vi "CRYTrigger advanced.vi"(0 "N sample":i32, 1 "N points":i32, 5 "Slope":u32(slide), 7 "Signal":dbl[](array[numeric]), 9 "Pretrigger ms":dbl format="%.6f", 11 "Trigger level (counts)":i32 format="%.3f", 12 "dt":dbl format="%.6f", 13 "Free run":bool, 15 "Reset buffer":bool) -> (4 "Triggered signal":dbl[](array[numeric]), 6 "Triggered":bool)   [LabVIEW 2013]
panel:
  out "x+y 2":i32
  out "x+y":i32
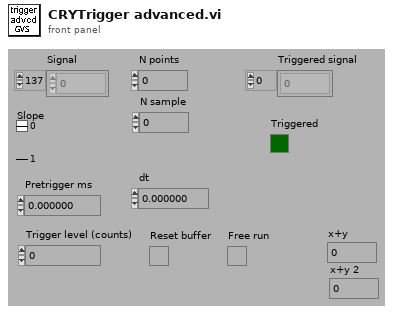
[diagram p1: front panel]
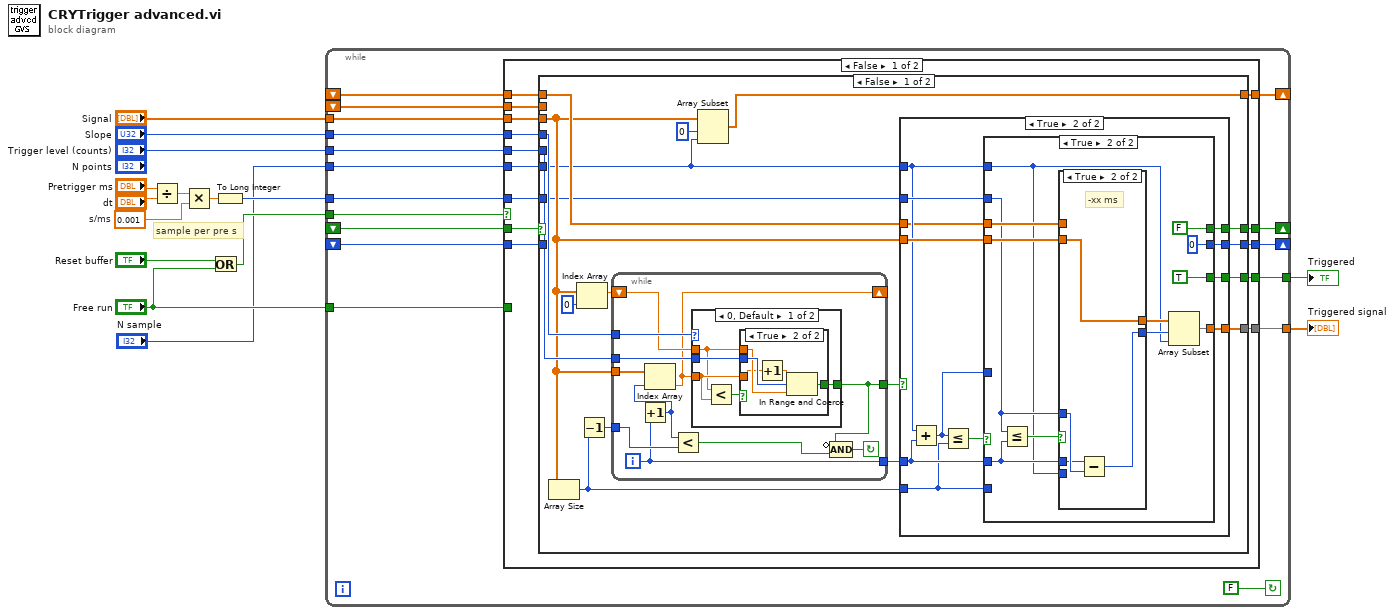
[diagram p0: block diagram]
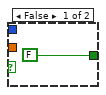
[diagram p2: hidden frame]
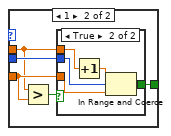
[diagram p3: hidden frame]
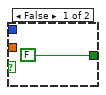
[diagram p4: hidden frame]
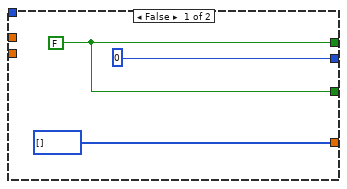
[diagram p5: hidden frame]
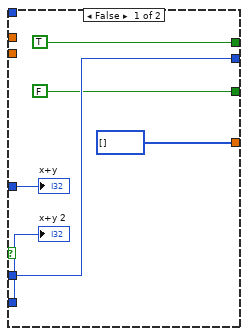
[diagram p6: hidden frame]
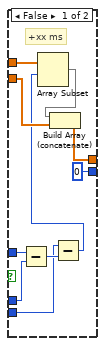
[diagram p7: hidden frame]
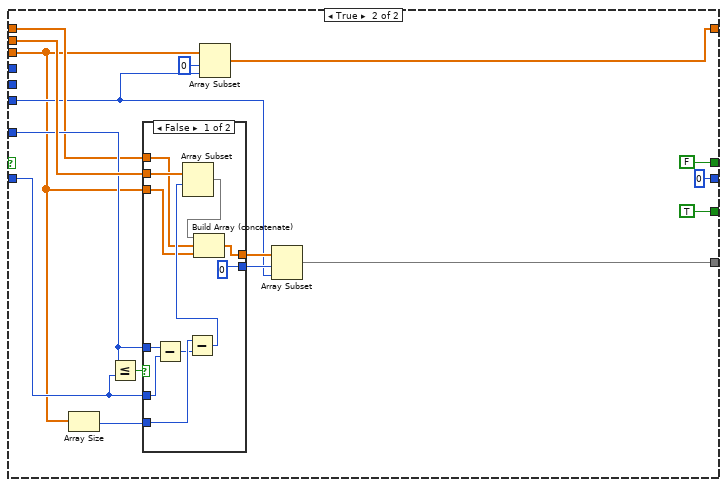
[diagram p8: hidden frame]
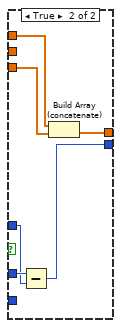
[diagram p9: hidden frame]
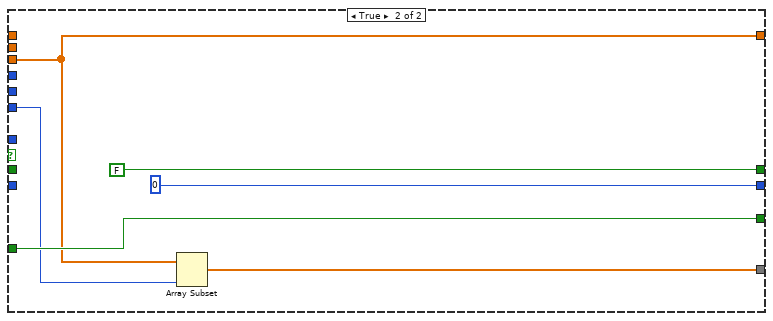
[diagram p10: hidden frame]
diagram:
  w10 = 0.001  # s/ms
  # "sample per pre s"
  n1 = Divide(x="Pretrigger ms", y="dt") -> (x/y=w9:dbl)
  n2 = Multiply(x=w9, y=w10) -> (x*y=w8:dbl)
  n3 = Or(x="Reset buffer", y="Free run") -> (x .or. y?=w4:bool)
  n4 = To Long Integer(number=w8) -> (32bit integer=w7:i32)
  n5 = while {
    tunnel: "Free run" -> [w19]
    shift-left: _ -> [w20]
    tunnel: w7 -> [w21]
    tunnel: "N sample" -> [w22]
    tunnel: "Trigger level (counts)" -> [w23]
    tunnel: "Slope" -> [w24]
    shift-left: _ -> [w25]
    shift-right: [w26] -> _
    tunnel: [w27] -> w2
    tunnel: [w28] -> w15
    tunnel: "Signal" -> [w16]
    tunnel: w4 -> [w32]
    shift-left: _ -> [w29]
    shift-right: [w30] -> _
    shift-left: _ -> [w17]
    shift-right: [w31] -> _
    stop <- FALSE continue-if-true
    n6 = case shown="False" w32 {
      tunnel: [w37 w180] -> w31
      tunnel: w16 -> [w44 w180]
      tunnel: [w40 FALSE] -> w30
      tunnel: w29 -> [w46 _]
      tunnel: w17 -> [w45 _]
      tunnel: [w39 w181] -> w28
      tunnel: [w41 w179] -> w27
      tunnel: [w38 0] -> w26
      tunnel: w25 -> [w33 _]
      tunnel: w24 -> [w43 _]
      tunnel: w23 -> [w42 _]
      tunnel: w22 -> [w36 w178]
      tunnel: w21 -> [w35 _]
      tunnel: w20 -> [w34 _]
      tunnel: w19 -> [_ w181]
      frame False {
        n7 = case shown="False" w46 {
          tunnel: w45 -> [w53 w149]
          tunnel: w44 -> [w52 w145]
          tunnel: w43 -> [w62 _]
          tunnel: w42 -> [w61 _]
          tunnel: [w59 w150] -> w41
          tunnel: [w58 FALSE] -> w40
          tunnel: [w57 TRUE] -> w39
          tunnel: [w56 0] -> w38
          tunnel: [w51 w146] -> w37
          tunnel: w36 -> [w50 w148]
          tunnel: w35 -> [w48 w151]
          tunnel: w34 -> [_ w153]
          tunnel: w33 -> [_ w154]
          frame False {
            n8 = Array Size(array=w52) -> (size(s)=w54:i32)
            n9 = Index Array(array=w52, index=0) -> (element=w63:dbl)
            n10 = Decrement(x=w54) -> (x-1=w64:i32)
            n11 = while {
              tunnel: [w65] -> w55
              tunnel: [w66] -> w60
              tunnel: w61 -> [w72]
              tunnel: w62 -> [w74]
              shift-left: w63 -> [w73]
              shift-right: [w71] -> _
              tunnel: w64 -> [w69]
              tunnel: w52 -> [w75]
              i -> [w65]
              stop <- w67 continue-if-true
              n12 = Increment(x=w65) -> (x+1=w70:i32)
              n13 = Index Array(array=w75, index=w70) -> (element=w71:dbl)
              n14 = Less?(x=w70, y=w69) -> (x < y?=w68:bool)
              n15 = case shown="0, Default" w74 {
                tunnel: w73 -> [w77 w88]
                tunnel: w72 -> [w79 w90]
                tunnel: w71 -> [w78 w89]
                tunnel: [w76 w87] -> w66
                frame 0, Default {
                  n16 = Less?(x=w77, y=w78) -> (x < y?=w80:bool)
                  n17 = case shown="True" w80 {
                    tunnel: w79 -> [_ w86]
                    tunnel: w78 -> [_ w83]
                    tunnel: w77 -> [_ w85]
                    tunnel: [FALSE w84] -> w76
                    frame False {
                    }
                    frame True {
                      n18 = Increment(x=w83) -> (x+1=w82:dbl)
                      n19 = In Range and Coerce(upper limit=w82, x=w86, lower limit=w85) -> (In Range?=w84:bool)  [unwired: 1 out]
                    }
                  }
                }
                frame 1 {
                  n20 = Greater?(x=w88, y=w89) -> (0:w91:bool)
                  n21 = case shown="True" w91 {
                    tunnel: w90 -> [_ w97]
                    tunnel: w89 -> [_ w95]
                    tunnel: w88 -> [_ w94]
                    tunnel: [FALSE w96] -> w87
                    frame False {
                    }
                    frame True {
                      n22 = Increment(x=w94) -> (x+1=w93:dbl)
                      n23 = In Range and Coerce(upper limit=w93, x=w97, lower limit=w95) -> (In Range?=w96:bool)  [unwired: 1 out]
                    }
                  }
                }
              }
              n24 = Compound Arithmetic op=AND(invert w66, w68) -> (w67:bool)
            }
            n25 = Array Subset(array=w52, index=0, length=w50) -> (w51:dbl[])
            n26 = case shown="True" w60 {
              tunnel: [i32[] [] ("Triggered signal") w107] -> w59
              tunnel: [w99 w111] -> w58
              tunnel: [w99 w108] -> w57
              tunnel: [0 w110] -> w56
              tunnel: w50 -> [_ w104]
              tunnel: w55 -> [_ w109]
              tunnel: w54 -> [_ w102]
              tunnel: w52 -> [_ w106]
              tunnel: w48 -> [_ w105]
              tunnel: w53 -> [_ w103]
              frame False {
                w99 = FALSE
              }
              frame True {
                n27 = Add(x=w104, y=w109) -> (x+y=w101:i32)
                n28 = Less Or Equal?(x=w101, y=w102) -> (x <= y?=w112:bool)
                n29 = case shown="True" w112 {
                  tunnel: [TRUE FALSE] -> w111
                  tunnel: [w117 0] -> w110
                  tunnel: w109 -> [w117 w126]
                  tunnel: [FALSE TRUE] -> w108
                  tunnel: [i32[] [] ("Triggered signal") w120] -> w107
                  tunnel: w106 -> [_ w125]
                  tunnel: w105 -> [_ w122]
                  tunnel: w104 -> [_ w119]
                  tunnel: w103 -> [_ w123]
                  tunnel: w102 -> [w113 _]
                  tunnel: w101 -> [w114 _]
                  frame False {
                    "x+y" <- w114
                    "x+y 2" <- w113
                  }
                  frame True {
                    n30 = Less Or Equal?(x=w122, y=w126) -> (x <= y?=w127:bool)
                    n31 = case shown="True" w127 {
                      tunnel: w126 -> [w135 w142]
                      tunnel: w122 -> [w140 w144]
                      tunnel: w125 -> [w138 w143]
                      tunnel: [w133 w143] -> w121
                      tunnel: [0 w141] -> w124
                      tunnel: w123 -> [w139 _]
                      tunnel: w119 -> [w131 _]
                      frame False {
                        # "+xx ms"
                        n32 = Subtract(x=w140, y=w135) -> (x-y=w136:i32)
                        n33 = Subtract(x=w131, y=w136) -> (x-y=w137:i32)
                        n34 = Array Subset(array=w139, index=w137) -> (w134:dbl[])  [unwired: 1 in]
                        n35 = Build Array (concatenate)(w134, w138) -> (w133:dbl[])
                      }
                      frame True {
                        # "-xx ms"
                        n36 = Subtract(x=w142, y=w144) -> (x-y=w141:i32)
                      }
                    }
                    n37 = Array Subset(array=w121, index=w124, length=w119) -> (w120:dbl[])
                  }
                }
              }
            }
          }
          frame True {
            n38 = Array Size(array=w145) -> (size(s)=w152:i32)
            n39 = Less Or Equal?(x=w151, y=w154) -> (x <= y?=w157:bool)
            n40 = case shown="False" w157 {
              tunnel: w154 -> [w170 w177]
              tunnel: w151 -> [w171 w176]
              tunnel: w153 -> [w163 _]
              tunnel: [w168 w172] -> w156
              tunnel: [0 w175] -> w155
              tunnel: w149 -> [w162 w173]
              tunnel: w152 -> [w167 _]
              tunnel: w145 -> [w161 w174]
              frame False {
                n41 = Subtract(x=w171, y=w170) -> (x-y=w166:i32)
                n42 = Subtract(x=w167, y=w166) -> (x-y=w165:i32)
                n43 = Array Subset(array=w163, index=w165) -> (w164:dbl[])  [unwired: 1 in]
                n44 = Build Array (concatenate)(w164, w162, w161) -> (w168:dbl[])
              }
              frame True {
                n45 = Subtract(x=w177, y=w176) -> (x-y=w175:i32)
                n46 = Build Array (concatenate)(w173, w174) -> (w172:dbl[])
              }
            }
            n47 = Array Subset(array=w145, index=0, length=w148) -> (w146:dbl[])
            n48 = Array Subset(array=w156, index=w155, length=w148) -> (w150:dbl[])
          }
        }
      }
      frame True {
        n49 = Array Subset(array=w180, length=w178) -> (w179:dbl[])  [unwired: 1 in]
      }
    }
  }
  "Triggered" <- w15
  "Triggered signal" <- w2
